vi "Solenoid Temp.vi"() -> ()   [LabVIEW 2018]
panel:
  out "Solenoid B Temp":dbl(slide) scale=0.0..100.0
  out "Solenoid A Temp":dbl(slide) scale=0.0..100.0
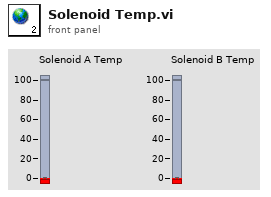
[diagram p1: front panel]
diagram:
